vi "UHR-Fleezers Control (fpga, with oscillation) - 10.3.vi"() -> ()   [LabVIEW 2013]
doc: "UHR-Fleezers Instrument Control Code (fpga)"
uses:
  <vilib>/Platform/TimedLoop/XDataNode/timing_clust.ctl
  <vilib>/Platform/TimedLoop/XDataNode/nitl_modes.ctl
  <vilib>/Platform/TimedLoop/XDataNode/wakeup.ctl
  <vilib>/rvi/eio/common/nirviEmuTemplateMethod_errors.vi
  <vilib>/rvi/Emulation/niFpgaSctlEmulationGetInTimedLoop.vi
  <vilib>/rvi/Emulation/niFpgaEmulationReportErrorSimple.vi
  <vilib>/rvi/Emulation/niFpgaGetClockAttributes.vi
  <vilib>/rvi/Emulation/niFpgaCriticalErrorInLSC.vi
  <vilib>/rvi/Emulation/niFpgaProcessEmulError.vi
  <vilib>/rvi/interface/RandomDataEmulation/nirviRandomDataFPGAFIFO.vi
  <vilib>/rvi/interface/RandomDataEmulation/niFpgaRandomDataHandleErrors.vi
  <vilib>/rvi/DataTransferAndStorage/Container/Common/niFpgaContainerExecOnDevCompGetState.vi
  <vilib>/rvi/Memory/Memory_Emulation/nirvimemoryFastEmulationFpgaImpl.vi
  <instcachedir>/0/nirvimemoryFastEmulationFpgaImpl_5FBAB50466BC4C939F684F8805638BFC.lvgen/nirvimemoryFastEmulationFpgaImpl_5FBAB50466BC4C939F684F8805638BFC_002.vi
  <vilib>/rvi/DataTransferAndStorage/Container/Common/niFpgaContainerGetUniqueNameForEmu.vi
  <vilib>/rvi/Memory/Memory_Emulation/niFpgaMemoryEmulationCacheClearOnFirstRun.vi
  <vilib>/rvi/Memory/Memory_Emulation/nirvimemoryEmulationManagerCache_MakeExclusive.vi
  <vilib>/rvi/Memory/Memory_Emulation/niFpgaMemoryEmulationValidateCache.vi
  <vilib>/rvi/Memory/Memory_Emulation/nirvimemoryEmulationManagerCache_ReleaseExclusive.vi
  <vilib>/rvi/Memory/Memory_Emulation/nirvimemoryEmulationManagerCache_InsertValue.vi
  <vilib>/Utility/error.llb/Clear Errors.vi
  <vilib>/rvi/Memory/Memory_Emulation/nirvimemoryEmulationManagerCache_SetValue.vi
  <vilib>/rvi/Emulation/niFpgaSctlEmulationResourceMgr.vi
  <vilib>/rvi/Memory/Memory_Emulation/nirvimemoryEmulationManagerCache_GetValue.vi
  <vilib>/Platform/TimedLoop/XDataNode/XDataNode.xnode
  <vilib>/eio/EIOMethodNode/EIOMethodNode.xnode
  <vilib>/eio/EIONode/EIONode.xnode
  <vilib>/rvi/DataTransferAndStorage/Container/XNode/niFpgaContainer.xnode
  <vilib>/rvi/interface/RandomDataEmulation/nirviRandomDataFpgaReadWriteTemplate.vi
  <vilib>/rvi/Memory/Memory_Emulation/niFpgaMemoryEmulationRefIn.vi
  <vilib>/addons/control/pid/fpga.llb/XNode/niFpgaPID.xnode
  <vilib>/Platform/TimedLoop/XDataNode/XDNodeRunTimeDep.lvlib
panel:
  out "Trap Pos FB Int-Norm Signal":fxp<+/-,16,1> format="%.16g"
  out "Trap Pos FB Int Signal":fxp<+/-,24,9> format="%.18g"
  in  "Tab Control":T1(tab)
  in  "AI1 X Scale":u16
  in  "Trap Pos FB Monitor T1 or T2":bool
  in  "Trap Pos FB Negate Action":bool
  in  "Trap Pos. FB SP":fxp<+/-,16,1>
  in  "Trap Pos. FB Reset":bool
  in  "Trap Pos to FIFO":bool
  in  "AI1 Sets to FIFO":T2={"Set 1"=TRUE, "Set 2"=TRUE, "Set 3"=FALSE}
  in  "N of AI1 Int Acq Sets":i16=2 min=1 max=3 step=1
  out "AI Late Counter":u16
  in  "ai count":u32=400
  out "AI late?":bool
  in  "+ phase":bool
  in  "Phase count adjustment":i16
  out "Relative phase":i16
  in  "AI to FIFO":bool
  out "BD1 Frequency Out 1":u64
  out "BD1 Frequency Out 2":u64
  in  "Force feedback":bool
  out "AI1 X Set 1":fxp<+/-,16,1>
  in  "Trap Pos. FB Gains":T3={"proportional gain (Kc)"=0.0, "integral gain (Kc*Ts/Ti)"=10.0, "derivative gain (Kc*Td/Ts)"=0.0} {"proportional gain (Kc)" format="%.11g"; "integral gain (Kc*Ts/Ti)" format="%.11g"; "derivative gain (Kc*Td/Ts)" format="%.11g"}
  in  "Trap Pos. FB Range":T4={"output high"=0.999969482421875, "output low"=-1.0}
  in  "Trap Pos. FB Mult Factor":i64=2
  in  "Trap Pos. FB Offset Factor":i64
  out "AI1 X Set 2":fxp<+/-,16,1>
  out "Trap Pos FB Action":i64
  out "Trap Pos FIFO Timeout":u16
  out "Trap AI FIFO Timeout":u16
  in  "Trap FIFO Set Timeout":i32
  in  "Trap Pos FB Int Count":u16=100
  in  "Tab Control 2":T5(tab)
  in  "Swap F1 and F2":bool
  in  "Freq or Amp switch first":bool=TRUE
  in  "Cont. Scan":bool
  in  "Abort scan":bool
  in  "Cycles per step":u64
  in  "Scan BD":bool
  in  "Number of scans":u16
  in  "Scan steps":u64
  in  "Scan freq.  increment":i64
  out "Scanning":bool
  in  "Start scan":bool
  in  "OSK Bd 1":bool
  in  "Reset Bd 1":bool
  in  "RD":bool
  in  "PMODE":bool
  in  "OSK Bd 2":bool
  in  "Reset Bd 2":bool
  in  "Direct RF Box \nCommunication":bool
  in  "Data BD 2":u8 format="%08b"
  in  "Data BD 1":u8 format="%08b"
  in  "Address":u8 format="%02x"
  in  "Update Data":bool
  in  "FPGA Controls\n RF Box":bool
  in  "Number Interlace Cycles":u8=2 min=1 max=3
  in  "Interlace Off Parameters":u8=1 min=1 max=3
  in  "Interlace ON/OFF":bool
  out "DIO Relative phase":i16
  in  "Phase count adjustment (DIO)":i16
  in  "+ phase (DIO)":bool
  out "DIO Late Counter":u16
  out "DIO Late?":bool
  in  "DIO count 1 (ticks)":u32=400
  in  "DIO count 2 (ticks)":u32=400
  in  "DIO count 3 (ticks)":u32=400
  out "AI2 Y Sum Set 2":i16
  out "AI2 Y Sum Set 1":i16
  in  "FB Gains Set 1":T6={"proportional gain (Kc)"=10, "integral gain (Kc*Ts/Ti)"=5, "derivative gain (Kc*Td/Ts)"=0}
  in  "FB Setpoint Set 1":i16 min=0 step=1
  in  "FB Reset Set 1":bool
  in  "FB On/Off Set 1":bool
  in  "FB Reset Set 2":bool
  in  "FB On/Off Set 2":bool
  in  "FB Setpoint Set 2":i16 min=0 step=1
  in  "FB Gains Set 2":T6={"proportional gain (Kc)"=10, "integral gain (Kc*Ts/Ti)"=5, "derivative gain (Kc*Td/Ts)"=0}
  in  "FB output range 2":cluster{"output high":i16, "output low":i16}={"output high"=3000, "output low"=0}
  in  "FB output range 1":cluster{"output high":i16, "output low":i16}={"output high"=3000, "output low"=0}
  out "Scan I":u64
  in  "Amp switch delay":u16=5
  in  "Freq switch delay":u16
  in  "Osc trap cont.":bool
  in  "Osc traps":bool
  in  "Initiate trap osc":bool
  in  "Trap osc period (pts)":i16
  in  "N trap osc periods":i16
  in  "Trap 1 osc enable":bool
  in  "Trap 2 osc enable":bool
  in  "Ready Write":bool
  in  "Data":i64
  in  "Address 2":u32
  in  "BD 2 Amplitude 1":u16
  in  "BD 1 Amplitude 1":u16
  in  "BD 2 Frequency 1":u64
  in  "BD 1 Frequency 1":u64
  in  "BD 2 Amplitude 2":u16
  in  "BD 1 Amplitude 2":u16
  in  "BD 2 Frequency 2":u64
  in  "BD 1 Frequency 2":u64
  in  "BD 2 Amplitude 3":u16
  in  "BD 1 Amplitude 3":u16
  in  "BD 2 Frequency 3":u64
  in  "BD 1 Frequency 3":u64
  out "Numeric":i32
  out "AO2 2":i16
  out "AO1 2":i16
  in  "1D or 2D Scan?":bool
  in  "Abort scan (MCL)":bool
  in  "MCL Scan Axis":bool
  in  "Cont. Scan (MCL)":bool
  out "Scan I (MCL)":u64
  in  "Number of scans (MCL)":u16
  out "Scanning MCL":bool
  in  "Scan steps (MCL)":u64
  in  "Cycles per step (MCL)":u64
  in  "Scan freq.  increment (MCL)":i16
  in  "Start scan (MCL)":bool
  in  "AO2":i16
  in  "AO1":i16
  out "MCL Late Counter":u16
  out "MCL Late?":bool
  in  "MCL count":u32=800
  out "MCL Relative Phase":i16
  in  "Phase count adjustment (MCL)":i16
  in  "+ phase (MCL)":bool
  in  "APD Gate Operating Mode":u8 max=2 step=1
  in  "Invert APD Gate":bool
  in  "APD Gate OFF Count":u32=100
  in  "APD Gate ON Count":u32=300
  out "APD 1 Gate Late Counter":u16
  out "APD 1 Gate Late?":bool
  out "APD 1 Gate Relative Phase":i16
  in  "Phase count adjustment (APD 1 Gate)":i16
  in  "+ phase (APD 1 Gate)":bool
  out "APD 2 Counts 0":u32
  out "APD 2 Counts 1":u32
  out "APD 1 Counts 0":u32
  out "APD 1 Counts 1":u32
  out "APD1 out state":bool
  in  "APD 2 AO scale factor":i16=1
  in  "APD 1 AO scale factor":i16=1
  in  "APD to FIFO":bool
  in  "APD Acq Rate Count":u32=20000000
  out "APD Acq Late Counter":u16
  out "APD Acq Late?":bool
  out "APD Acq Relative Phase":i16
  in  "Phase Count Adjustment (APD Acq)":i16
  in  "+ phase (APD Acq)":bool
  in  "Phase count adjustment (APD 2 Gate)":i16
  out "APD 2 Gate Late Counter":u16
  out "APD 2 Gate Late?":bool
  out "APD 2 Gate Relative Phase":i16
  in  "+ phase (APD 2 Gate)":bool
  out "APD2 out state":bool
  in  "Green Filter Flipper":bool
  out "Green FB Signals":T7
  in  "Green FB Count":u32=1200
  out "Green Late Counter":u16
  out "Green FB Late?":bool
  out "Green FB Relative Phase":i16
  in  "Phase count adjustment (Green FB)":i16=10
  in  "+ phase (Green FB)":bool
  out "Green FB Sum":i16
  in  "Green int current ON count adj":u32=150
  in  "Current Out":u16=30000
  in  "Green FB On/Off":bool
  in  "Green FB Setpoint":i16=250 min=0 step=1
  in  "Green FB Gains":T6={"proportional gain (Kc)"=10, "integral gain (Kc*Ts/Ti)"=5, "derivative gain (Kc*Td/Ts)"=0}
  in  "Green FB Reset":bool
  in  "Operating Mode 2":u8=2 max=2 step=1
  in  "Invert GI 2":bool
  in  "Green interlace OFF count 2":u32=900
  in  "Green interlace ON count 2":u32=300
  out "GI Late Counter 2":u16
  out "GI Late? 2":bool
  out "GI Relative phase 2":i16
  in  "Phase count adjustment (GI) 2":i16=20
  in  "+ phase (GI) 2":bool
  in  "Green interlace OFF count":u32=100
  out "GI Relative phase":i16
  in  "Phase count adjustment (GI)":i16
  in  "+ phase (GI)":bool
  out "GI Late?":bool
  in  "Green interlace ON count":u32=300
  out "GI Late Counter":u16
  in  "Invert GI":bool
  in  "Operating Mode":u8 max=2 step=1
  in  "Chassis2/Mod4/AO1":u16
  # "Oscillate Traps\n(e.g., for forced calibration)"
  # "Raster Scan AOD"
  # "Only one of these can be on\nat a time:"
  # "1 (X)"
  # "2 (Y)"
  # "IR Intensity Feedback (RF BD 1)"
  # "AO1 (Y)"
  # "2D"
  # "1D"
  # "AO2 (X)"
  # "APD AO for aligning"
  # "Detection Loop"
  # "Green fluorescent laser digital gate interlacing loop"
  # "0 Forced ON\n1 Forced OFF\n2 Interlacing"
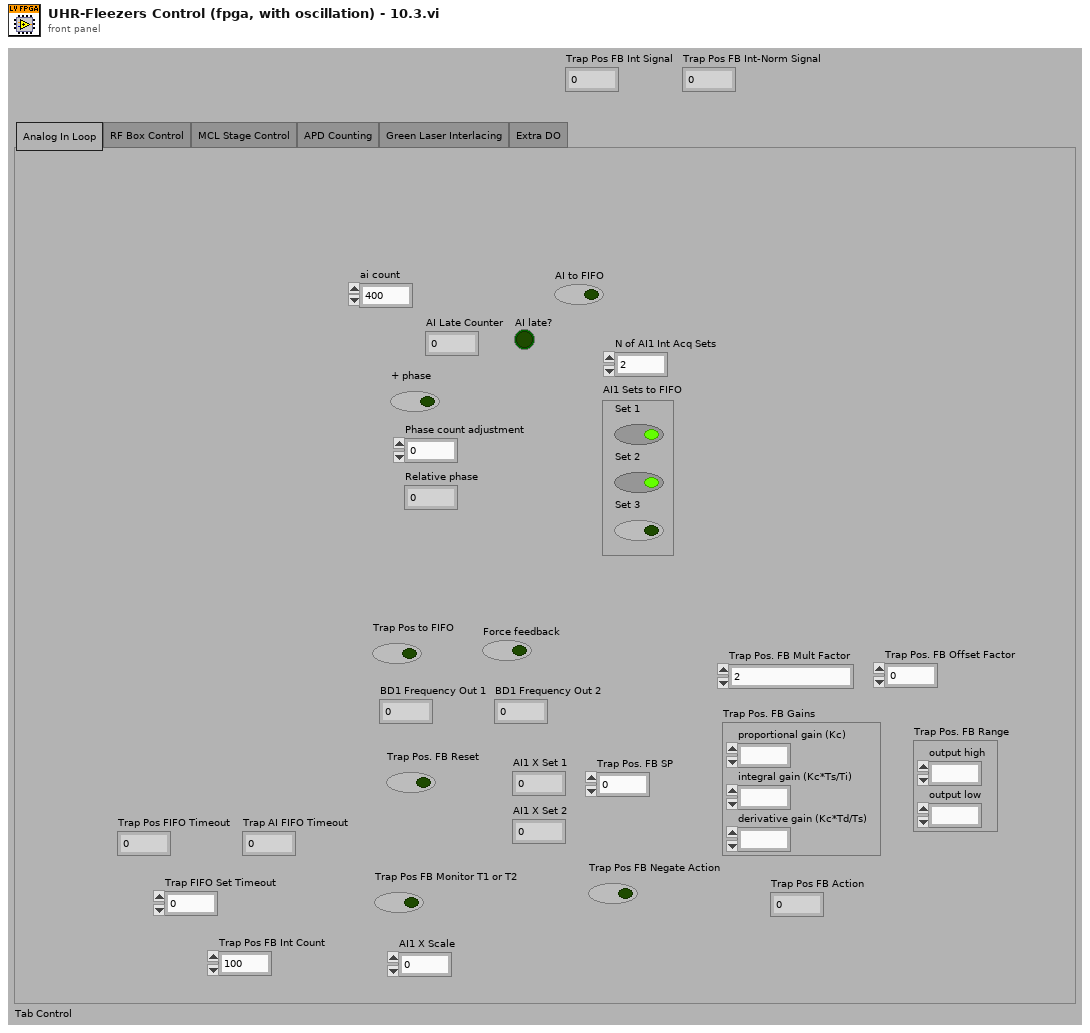
[diagram p1: front panel]
types:
  T1 = enum32{"Analog In Loop", "RF Box Control", "MCL Stage Control", "APD Counting", "Green Laser Interlacing", "Extra DO"}
  T2 = cluster{"Set 1":bool, "Set 2":bool, "Set 3":bool}
  T3 = cluster{"proportional gain (Kc)":fxp<+/-,16,8>, "integral gain (Kc*Ts/Ti)":fxp<+/-,16,8>, "derivative gain (Kc*Td/Ts)":fxp<+/-,16,8>}
  T4 = cluster{"output high":fxp<+/-,16,1>, "output low":fxp<+/-,16,1>}
  T5 = enum32{"Controls", "Interlacing Frequency and Amplitude Values"}
  T6 = cluster{"proportional gain (Kc)":i16, "integral gain (Kc*Ts/Ti)":i16, "derivative gain (Kc*Td/Ts)":i16}
  T7 = cluster{"Green FB Ch 0":i16, "Green FB Ch 1":i16, "Green FB Ch 2":i16}
  T8 = typedef "XDNodeRunTimeDep.lvlib/timing_clust.ctl" = cluster{"Expected End [f-1]":u64, "Actual End [f-1]":u64, "Finished Late? [f-1]":bool, "Expected End [i-1]":u64, "Actual End [i-1]":u64, "Finished Late? [i-1]":bool, "Expected Start [i]":u64, "Actual Start [i]":u64, "Expected Start [f]":u64, "Actual Start [f]":u64, "Source Name":string, "Structure Name":string, "Period":i64, "Deadline":i64, "Offset":i64, "Start":i64, "Priority":i32, "Timeout":i32, "Mode":T9, "Wakeup Reason":T10, "Error":errorcluster, "Source Type":string, "Secondary Source Type":string, "Global End Time":u64, "Global Start Time":u64, "Frame Duration":u64, "Iteration Duration":u64, "Assigned CPU":i32, "I/O Scan Engine Mode":u32}
  T9 = typedef "XDNodeRunTimeDep.lvlib/nitl_modes.ctl" = enum32{"No Change", "Process missed periods, maintain original phase", "Discard missed periods, maintain original phase", "Process missed periods, ignore original phase", "Discard missed periods, ignore original phase"}
  T10 = typedef "XDNodeRunTimeDep.lvlib/wakeup.ctl" = enum32{"Normal", "Aborted", "Asynchronous wakeup", "Timing source error", "Timed loop error", "Timeout"}
  T11 = cluster{"Chassis2/Mod2/AI0":i16, "Chassis2/Mod2/AI1":i16, "Chassis2/Mod2/AI2":i16}
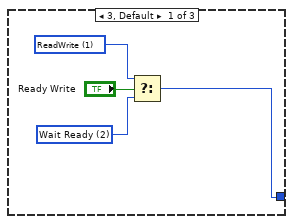
[diagram p2: hidden frame]
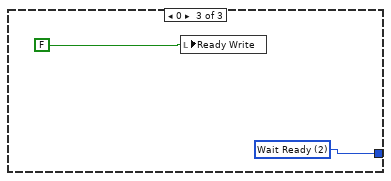
[diagram p3: hidden frame]
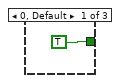
[diagram p4: hidden frame]
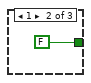
[diagram p5: hidden frame]
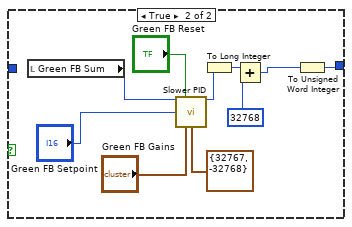
[diagram p6: hidden frame]
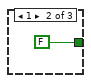
[diagram p7: hidden frame]
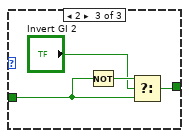
[diagram p8: hidden frame]
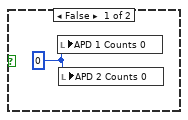
[diagram p9: hidden frame]
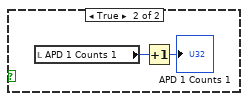
[diagram p11: hidden frame]
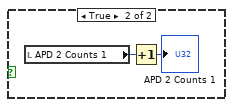
[diagram p12: hidden frame]
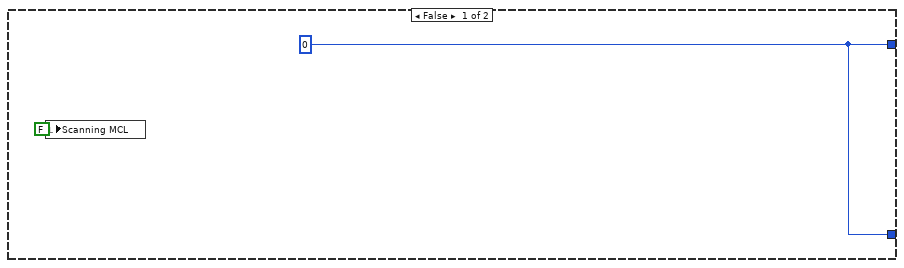
[diagram p13: hidden frame]
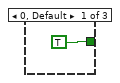
[diagram p14: hidden frame]
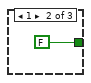
[diagram p15: hidden frame]
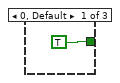
[diagram p16: hidden frame]
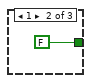
[diagram p17: hidden frame]
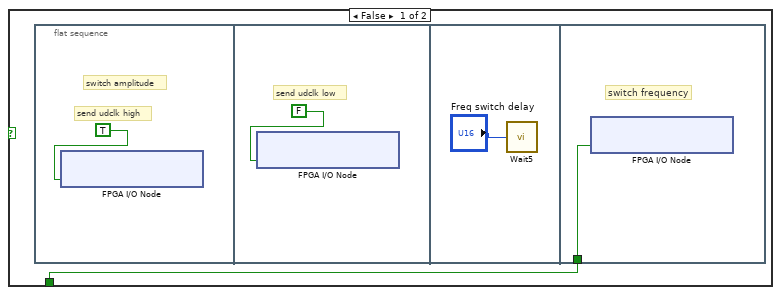
[diagram p20: hidden frame]
diagram:
  w1 = i16 2 items=["UnSet Ready", "ReadWrite", "Wait Ready"]
  w4 = FALSE
  # "timing array current index"
  # "timing array"
  # "timing counter (phase adjusted here)"
  # "late counter"
  n1 = flat-sequence "FPGA initialization to do before running any of the loops" {
    tunnel: [u32 0 ("DIO count 3 (ticks)")] -> w3
    tunnel: [w11] -> _
    frame #0 {
      # "Start up expansion chassis early\nto avoid delays later"
      # "This pin controls udclk on the RF boards.\nWhen initially configuring the boards, this pin needs to be\nconfigured as a high impedance input.  Later it will be switched\nto an output."
      # "Initial setting of DIO data and \naddress to low (before reset).  \nThis needs to happen before the other\ncontrol method loops execute."
      n2 = xnode "FPGA I/O Node"("Connector1/DIO0"=FALSE, "Connector1/DIO1"=FALSE, "Connector1/DIO2"=FALSE, "Connector1/DIO3"=FALSE, "Connector1/DIO4"=FALSE, "Connector1/DIO5"=FALSE, "Connector1/DIO6"=FALSE, "Connector1/DIO7"=FALSE, "Connector1/DIO8"=FALSE, "Connector1/DIO9"=FALSE, "Connector1/DIO10"=FALSE, "Connector1/DIO11"=FALSE, "Connector1/DIO12"=FALSE, "Connector1/DIO13"=FALSE, "Connector1/DIO15"=FALSE, "Connector1/DIO20"=FALSE, "Connector1/DIO21"=FALSE, "Connector1/DIO22"=FALSE, "Connector1/DIO23"=FALSE, "Connector1/DIO24"=FALSE, "Connector1/DIO25"=FALSE, "Connector1/DIO26"=FALSE, "Connector1/DIO27"=FALSE, "Connector1/DIO14"=FALSE) -> ()  [unwired: 24 in, 24 out]
      n3 = xnode "FPGA I/O Method Node"("Enable"=FALSE) -> ()  [unwired: 1 in, 1 out]
      n4 = xnode "FPGA I/O Node"("Chassis2/Mod1/AO0"=u16 0 ("Chassis2/Mod4/AO0")) -> ("Chassis2/Mod2/AI0"=w11:i16)  [unwired: 2 in, 2 out]
    }
  }
  n5 = node-c288() -> (w6:T8)  [unwired: 1 in]
  n6 = timed-loop "RF box board DIO control: control bits" {
    timing: w6 -> [_]
    timing-out: [_] -> w5
    tunnel: [w39] -> _
    tunnel: w3 -> [w39]
    stop <- FALSE stop-if-true
    n7 = xnode "FPGA I/O Node"("Connector1/DIO16"="RD", "Connector1/DIO17"="PMODE", "Connector1/DIO18"="OSK Bd 1", "Connector1/DIO19"="Reset Bd 1", "Connector1/DIO28"="OSK Bd 2", "Connector1/DIO29"="Reset Bd 2") -> ()  [unwired: 6 in, 6 out]
  }
  n8 = local read "AO1"() -> (w8:i16)
  n9 = local read "AO2"() -> (w7:i16)
  n10 = while "APD 1 Counter" {
    tunnel: w3 -> [_]
    stop <- FALSE stop-if-true
    n11 = flat-sequence {
      frame #0 {
        n12 = xnode "FPGA I/O Method Node"("FPGA I/O In"=refnum<k21> "Connector0/DIO0" ("APD 1 DO"), "Timeout"=-1) -> ()  [unwired: 2 out]
      }
      frame #1 {
        n13 = local read "APD1 out state"() -> (w52:bool)
        n14 = case shown="False" w52 {
          frame False {
            n15 = local read "APD 1 Counts 0"() -> (w54:u32)
            n16 = Increment(x=w54) -> (x+1=→"APD 1 Counts 0":u32)
          }
          frame True {
            n17 = local read "APD 1 Counts 1"() -> (w56:u32)
            n18 = Increment(x=w56) -> (x+1=→"APD 1 Counts 1":u32)
          }
        }
      }
    }
  }
  n19 = while "APD 2 Counter" {
    tunnel: w3 -> [_]
    stop <- FALSE stop-if-true
    n20 = flat-sequence {
      frame #0 {
        n21 = xnode "FPGA I/O Method Node"("FPGA I/O In"=refnum<k21> "Connector0/DIO1" ("APD 2 DO"), "Timeout"=-1) -> ()  [unwired: 2 out]
      }
      frame #1 {
        n22 = local read "APD2 out state"() -> (w60:bool)
        n23 = case shown="False" w60 {
          frame False {
            n24 = local read "APD 2 Counts 0"() -> (w62:u32)
            n25 = Increment(x=w62) -> (x+1=→"APD 2 Counts 0":u32)
          }
          frame True {
            n26 = local read "APD 2 Counts 1"() -> (w64:u32)
            n27 = Increment(x=w64) -> (x+1=→"APD 2 Counts 1":u32)
          }
        }
      }
    }
  }
  n28 = while "Control Additional IO (Green laser flip mount)" {
    stop <- FALSE stop-if-true
    n29 = xnode "FPGA I/O Node"("Connector0/DIO3"="Green Filter Flipper", "Chassis2/Mod1/AO1"="Chassis2/Mod4/AO1") -> ()  [unwired: 2 in, 2 out]
    n30 = call "Loop Timer2"("Count(Ticks)"=u32 40000 ("Extra DO Counts")) -> ()  [unwired: 1 out]
  }
  n31 = while "Handshake memory transfer for trap oscillation sin wave data" {
    shift-right: [w70] -> _
    shift-left: w1 -> [w71]
    stop <- FALSE stop-if-true
    # "Write"
    n32 = case shown="1" w71 {
      tunnel: [w74 w79 w80] -> w70
      frame 3, Default {
        w72 = i16 2 items=["UnSet Ready", "ReadWrite", "Wait Ready"]
        w73 = i16 1 items=["UnSet Ready", "ReadWrite", "Wait Ready"]
        n33 = Select(t=w73, s="Ready Write", f=w72) -> (s? t:f=w74:i16)
      }
      frame 1 {
        w79 = i16 0 items=["UnSet Ready", "ReadWrite", "Wait Ready"]
        n34 = xnode ("Memory Write")("Address"="Address 2", "Data"="Data", "Memory In"=refnum<k21> "Trap osc memory") -> ()  [unwired: 1 out]
      }
      frame 0 {
        w80 = i16 2 items=["UnSet Ready", "ReadWrite", "Wait Ready"]
        n35 = local write "Ready Write"(FALSE ("Ready Read")) -> ()
      }
    }
  }
  n36 = while "RF box board direct communication loop" {
    tunnel: w3 -> [_]
    stop <- FALSE stop-if-true
    n37 = case "Whether to use direct communication method (only use one method at a time)" shown="True" "Direct RF Box \nCommunication" {
      frame False {
      }
      frame True {
        n38 = case shown="True" "Update Data" {
          frame False {
          }
          frame True {
            n39 = flat-sequence {
              frame #0 {
                n40 = First Call?() -> (First Call?: T/F=w85:bool)
                n41 = case shown="True" w85 {
                  frame False {
                  }
                  frame True {
                    # "If first time data updated, be sure to set WR high\nbefore setting data and address bits."
                    n42 = flat-sequence {
                      frame #0 {
                        n43 = xnode "FPGA I/O Node"("Connector1/DIO15"=TRUE) -> ()  [unwired: 1 in, 1 out]
                      }
                      frame #1 {
                        n44 = call "Wait"("Count(Ticks)"=u8 40 ("DO Delay 3 (Ticks)")) -> ()  [unwired: 1 out]
                      }
                    }
                  }
                }
              }
              frame #1 {
                n45 = Number To Boolean Array(number="Address") -> (Boolean array=w134:bool[])
                n46 = Number To Boolean Array(number="Data BD 1") -> (Boolean array=w135:bool[])
                n47 = Number To Boolean Array(number="Data BD 2") -> (Boolean array=w104:bool[])
                n48 = Index Array(array=w135, index=7) -> (element=w119:bool)
                n49 = Index Array(array=w135, index=6) -> (element=w118:bool)
                n50 = Index Array(array=w135, index=5) -> (element=w117:bool)
                n51 = Index Array(array=w135, index=4) -> (element=w116:bool)
                n52 = Index Array(array=w135, index=3) -> (element=w115:bool)
                n53 = Index Array(array=w135, index=2) -> (element=w114:bool)
                n54 = Index Array(array=w135, index=1) -> (element=w113:bool)
                n55 = Index Array(array=w135, index=0) -> (element=w112:bool)
                n56 = Index Array(array=w134, index=5) -> (element=w111:bool)
                n57 = Index Array(array=w134, index=4) -> (element=w110:bool)
                n58 = Index Array(array=w134, index=3) -> (element=w109:bool)
                n59 = Index Array(array=w134, index=2) -> (element=w108:bool)
                n60 = Index Array(array=w134, index=1) -> (element=w107:bool)
                n61 = Index Array(array=w134, index=0) -> (element=w106:bool)
                n62 = Index Array(array=w104, index=7) -> (element=w95:bool)
                n63 = Index Array(array=w104, index=6) -> (element=w94:bool)
                n64 = Index Array(array=w104, index=5) -> (element=w93:bool)
                n65 = Index Array(array=w104, index=4) -> (element=w92:bool)
                n66 = Index Array(array=w104, index=3) -> (element=w91:bool)
                n67 = Index Array(array=w104, index=2) -> (element=w90:bool)
                n68 = Index Array(array=w104, index=1) -> (element=w89:bool)
                n69 = Index Array(array=w104, index=0) -> (element=w88:bool)
                n70 = xnode "FPGA I/O Node"("Connector1/DIO0"=w119, "Connector1/DIO1"=w118, "Connector1/DIO2"=w117, "Connector1/DIO3"=w116, "Connector1/DIO4"=w115, "Connector1/DIO5"=w114, "Connector1/DIO6"=w113, "Connector1/DIO7"=w112, "Connector1/DIO8"=w111, "Connector1/DIO9"=w110, "Connector1/DIO10"=w109, "Connector1/DIO11"=w108, "Connector1/DIO12"=w107, "Connector1/DIO13"=w106, "Connector1/DIO20"=w95, "Connector1/DIO21"=w94, "Connector1/DIO22"=w93, "Connector1/DIO23"=w92, "Connector1/DIO24"=w91, "Connector1/DIO25"=w90, "Connector1/DIO26"=w89, "Connector1/DIO27"=w88) -> ()  [unwired: 22 in, 22 out]
              }
              frame #2 {
                # "wait and then apply write signal"
                n71 = call "Wait2"("Count(Ticks)"=u8 40 ("DO Delay 1 (Ticks)")) -> ()  [unwired: 1 out]
              }
              frame #3 {
                # "sending bit low writes data to board buffer"
                n72 = xnode "FPGA I/O Node"("Connector1/DIO15"=FALSE) -> ()  [unwired: 1 in, 1 out]
              }
              frame #4 {
                # "wait then return write signal"
                n73 = call "Wait3"("Count(Ticks)"=u8 40 ("DO Delay 2 (Ticks)")) -> ()  [unwired: 1 out]
              }
              frame #5 {
                # "sending bit high makes ready to\nwrite more data"
                n74 = xnode "FPGA I/O Node"("Connector1/DIO15"=TRUE) -> ()  [unwired: 1 in, 1 out]
              }
            }
          }
        }
      }
    }
  }
  n75 = while "APD 2 Gating" {
    shift-right: [w145] -> _
    shift-left: w3 -> [w150]
    shift-right: [w144] -> _
    shift-left: w4 -> [w142]
    stop <- FALSE stop-if-true
    n76 = flat-sequence {
      tunnel: w150 -> [w153]
      tunnel: [w154] -> w148
      tunnel: [w153] -> w146
      tunnel: [w152] -> w143
      tunnel: w142 -> [w152]
      tunnel: [w157] -> w149
      tunnel: w148 -> [w157]
      tunnel: [w156] -> w147
      tunnel: w146 -> [w156]
      tunnel: w143 -> [w155]
      tunnel: [w175] -> w145
      tunnel: w149 -> [w186]
      tunnel: w147 -> [w184]
      tunnel: [w179] -> w144
      frame #0 {
        n77 = call "Loop Timer8"("Count(Ticks)"=w153) -> ("Tick Count(Ticks)"=w154:u32)
      }
      frame #1 {
        # "(need 4 channels/APD)"
        n78 = xnode "FPGA I/O Node"("Connector1/DIO26"=w155, "Connector1/DIO27"=w155, "Connector1/DIO22"=w155, "Connector1/DIO32"=w155, "Connector1/DIO34"=w155, "Connector1/DIO33"=w155, "Connector1/DIO35"=w155) -> ()  [unwired: 7 in, 7 out]
      }
      frame #2 {
        n79 = local read "APD Gate ON Count"() -> (w168:u32)
        n80 = local read "APD Gate OFF Count"() -> (w167:u32)
        n81 = feedback #1(TRUE) -> (w181:bool)
        n82 = feedback-in #2(w186) -> ()
        n83 = feedback #2(w186) -> (w169:u32)
        n84 = Not(x=w181) -> (.not. x?=w178:bool)
        n85 = feedback-in #1(w178) -> ()
        n86 = Subtract(x=w186, y=w169) -> (x-y=w185:u32)
        n87 = Select(t=w168, s=w178, f=w167) -> (s? t:f=w183:u32)
        n88 = Subtract(x=w185, y=w184) -> (x-y=w160:u32)
        n89 = Subtract(x=w183, y=w160) -> (x-y=w174:u32)
        n90 = Number To Boolean Array(number=w160) -> (Boolean array=w159:bool[])
        n91 = Or Array Elements(Boolean array=w159) -> (logical OR=w158:bool)
        "APD 2 Gate Late?" <- w158
        n92 = Boolean To (0,1)(Boolean="+ phase (APD 2 Gate)") -> (0, 1=w172:i16)
        n93 = Multiply(x=w172, y="Phase count adjustment (APD 2 Gate)") -> (x*y=w170:i16)
        n94 = Boolean To (0,1)(Boolean=w158) -> (0, 1=w165:i16)
        n95 = Add(x=w174, y=w170) -> (x+y=w175:u32)
        n96 = To Unsigned Word Integer(number=w165) -> (unsigned 16bit integer=w162:u16)
        n97 = feedback #3(i16 0) -> (w177:i16)
        n98 = Subtract(x=w177, y=w170) -> (x-y=w176:i16)
        "APD 2 Gate Relative Phase" <- w176
        n99 = feedback-in #3(w176) -> ()
        n100 = feedback #4(u16 0) -> (w163:u16)
        n101 = Add(x=w162, y=w163) -> (x+y=w161:u16)
        "APD 2 Gate Late Counter" <- w161
        n102 = feedback-in #4(w161) -> ()
        n103 = local read "APD Gate Operating Mode"() -> (w166:u8)
        n104 = case shown="2" w166 {
          tunnel: [TRUE FALSE w192] -> w179
          tunnel: w181 -> [_ _ w190]
          frame 0, Default {
          }
          frame 1 {
          }
          frame 2 {
            n105 = local read "Invert APD Gate"() -> (w189:bool)
            n106 = Not(x=w190) -> (.not. x?=w191:bool)
            n107 = Select(t=w191, s=w189, f=w190) -> (s? t:f=w192:bool)
          }
        }
      }
    }
  }
  n108 = while "APD 1 Gating" {
    shift-right: [w196] -> _
    shift-left: w3 -> [w201]
    shift-right: [w195] -> _
    shift-left: w4 -> [w193]
    stop <- FALSE stop-if-true
    n109 = flat-sequence {
      tunnel: w201 -> [w204]
      tunnel: [w205] -> w199
      tunnel: [w204] -> w197
      tunnel: [w203] -> w194
      tunnel: w193 -> [w203]
      tunnel: [w208] -> w200
      tunnel: w199 -> [w208]
      tunnel: [w207] -> w198
      tunnel: w197 -> [w207]
      tunnel: w194 -> [w206]
      tunnel: [w222] -> w196
      tunnel: w200 -> [w237]
      tunnel: w198 -> [w234]
      tunnel: [w226] -> w195
      frame #0 {
        n110 = call "Loop Timer7"("Count(Ticks)"=w204) -> ("Tick Count(Ticks)"=w205:u32)
      }
      frame #1 {
        # "(need 4 channels/APD)"
        n111 = xnode "FPGA I/O Node"("Connector0/DIO8"=w206, "Connector0/DIO9"=w206, "Connector0/DIO10"=w206, "Connector0/DIO11"=w206, "Connector0/DIO4"=w206, "Connector0/DIO5"=w206, "Connector0/DIO6"=w206, "Connector0/DIO7"=w206) -> ()  [unwired: 8 in, 8 out]
      }
      frame #2 {
        n112 = feedback #5(TRUE) -> (w229:bool)
        n113 = feedback-in #6(w237) -> ()
        n114 = feedback #6(w237) -> (w236:u32)
        n115 = Not(x=w229) -> (.not. x?=w225:bool)
        n116 = feedback-in #5(w225) -> ()
        n117 = Subtract(x=w237, y=w236) -> (x-y=w235:u32)
        n118 = Select(t="APD Gate ON Count", s=w225, f="APD Gate OFF Count") -> (s? t:f=w231:u32)
        n119 = Subtract(x=w235, y=w234) -> (x-y=w210:u32)
        n120 = Subtract(x=w231, y=w210) -> (x-y=w221:u32)
        n121 = Number To Boolean Array(number=w210) -> (Boolean array=w211:bool[])
        n122 = Or Array Elements(Boolean array=w211) -> (logical OR=w209:bool)
        "APD 1 Gate Late?" <- w209
        n123 = Boolean To (0,1)(Boolean="+ phase (APD 1 Gate)") -> (0, 1=w219:i16)
        n124 = Boolean To (0,1)(Boolean=w209) -> (0, 1=w216:i16)
        n125 = Multiply(x=w219, y="Phase count adjustment (APD 1 Gate)") -> (x*y=w217:i16)
        n126 = To Unsigned Word Integer(number=w216) -> (unsigned 16bit integer=w213:u16)
        n127 = Add(x=w221, y=w217) -> (x+y=w222:u32)
        n128 = feedback #7(i16 0) -> (w224:i16)
        n129 = Subtract(x=w224, y=w217) -> (x-y=w223:i16)
        "APD 1 Gate Relative Phase" <- w223
        n130 = feedback-in #7(w223) -> ()
        n131 = feedback #8(u16 0) -> (w214:u16)
        n132 = Add(x=w213, y=w214) -> (x+y=w212:u16)
        "APD 1 Gate Late Counter" <- w212
        n133 = feedback-in #8(w212) -> ()
        n134 = case shown="2" "APD Gate Operating Mode" {
          tunnel: [TRUE FALSE w243] -> w226
          tunnel: w229 -> [_ _ w240]
          frame 0, Default {
          }
          frame 1 {
          }
          frame 2 {
            n135 = Not(x=w240) -> (.not. x?=w242:bool)
            n136 = Select(t=w242, s="Invert APD Gate", f=w240) -> (s? t:f=w243:bool)
          }
        }
      }
    }
  }
  n137 = while "DAQ AI set 1" {
    shift-right: [w244] -> _
    shift-left: w3 -> [w249]
    stop <- FALSE stop-if-true
    n138 = flat-sequence {
      tunnel: w249 -> [w259]
      tunnel: [w260] -> w247
      tunnel: [w259] -> w246
      tunnel: [w270] -> w257
      tunnel: [w269] -> w256
      tunnel: [w268] -> w255
      tunnel: [w267] -> w254
      tunnel: [w266] -> w253
      tunnel: [w265] -> w252
      tunnel: [w264] -> w251
      tunnel: [w263] -> w250
      tunnel: [w262] -> w248
      tunnel: w247 -> [w262]
      tunnel: w246 -> [w261]
      tunnel: [w261] -> w245
      tunnel: [w299] -> w244
      tunnel: w257 -> [w327]
      tunnel: w256 -> [w291]
      tunnel: w255 -> [w292]
      tunnel: w254 -> [w326]
      tunnel: w253 -> [w315]
      tunnel: w252 -> [w314]
      tunnel: w251 -> [w313]
      tunnel: w250 -> [w312]
      tunnel: w248 -> [w309]
      tunnel: w245 -> [w306]
      frame #0 {
        n139 = call "Loop Timer3"("Count(Ticks)"=w259) -> ("Tick Count(Ticks)"=w260:u32)
      }
      frame #1 {
        # "detection \nlaser qpd"
        # "sum"
        # "x"
        # "y"
        # "1064 int\nfeedback qpd"
        # "sum"
        # "x"
        # "traps\nqpd"
        # "sum"
        # "y"
        # "x"
        n140 = xnode "FPGA I/O Node"("Connector1/DIO31"=TRUE ("Connector1/DIO33")) -> ("Connector0/AI0"=w270:i16, "Connector0/AI1"=w269:i16, "Connector0/AI2"=w268:i16, "Connector0/AI3"=w267:i16, "Connector0/AI4"=w266:i16, "Connector0/AI5"=w265:i16, "Connector0/AI6"=w264:i16, "Connector0/AI7"=w263:i16)  [unwired: 9 in, 9 out]
      }
      frame #2 {
        w295 = FALSE ("AI to FIFO")
        # "only write specified sets (1 and 2 usually) to FIFO \nif AI to FIFO is true"
        # "Adjust phase after data acquired if button pressed"
        n141 = feedback #9(i16 1) -> (w319:i16)
        n142 = Increment(x=w319) -> (x+1=w325:i16)
        n143 = Scale By Power Of 2(n="AI1 X Scale", x=w291) -> (x*2^n=w289:i16)
        n144 = Greater?(x=w325, y="N of AI1 Int Acq Sets") -> (0:w322:bool)
        n145 = Divide(x=w289, y=w292) -> (x/y=w288:fxp<+/-,16,1>)
        n146 = Select(t=i16 1, s=w322, f=w325) -> (s? t:f=w324:i16)
        n147 = feedback-in #9(w324) -> ()
        n148 = feedback #10(w295) -> (w293:bool)
        n149 = feedback #11(w295) -> (w311:bool)
        n150 = case shown="1, Default" w319 {
          tunnel: w292 -> [w349 w357 _]
          tunnel: "AI1 Sets to FIFO" -> [w353 w361 w367]
          tunnel: [w352 w360 w366] -> w316
          tunnel: ["AI to FIFO" w359 w365] -> w310
          tunnel: w311 -> [_ w359 w365]
          tunnel: ["Trap Pos to FIFO" w358 w364] -> w294
          tunnel: w293 -> [_ w358 w364]
          tunnel: w288 -> [w348 w356 _]
          tunnel: [w347 w354 FALSE] -> w275
          tunnel: [w346 w355 u64 0 ("BD1 Frequency Out 2")] -> w274
          frame 1, Default {
            n151 = Unbundle By Name(w353) -> ("Set 1"=w352:bool)
            n152 = local read "BD1 Frequency Out 1"() -> (w346:u64)
            n153 = Compound Arithmetic op=AND("Trap Pos to FIFO", w352, "AI to FIFO") -> (w347:bool)
            "AI2 Y Sum Set 1" <- w349
            "AI1 X Set 1" <- w348
          }
          frame 2 {
            n154 = Unbundle By Name(w361) -> ("Set 2"=w360:bool)
            n155 = local read "BD1 Frequency Out 2"() -> (w355:u64)
            n156 = Compound Arithmetic op=AND(w358, w360, w359) -> (w354:bool)
            "AI2 Y Sum Set 2" <- w357
            "AI1 X Set 2" <- w356
          }
          frame 3 {
            n157 = Unbundle By Name(w367) -> ("Set 3"=w366:bool)
          }
        }
        n158 = And(x=w316, y=w310) -> (x .and. y?=w318:bool)
        n159 = feedback-in #10(w294) -> ()
        n160 = case shown="True" w318 {
          tunnel: w327 -> [_ w381]
          tunnel: w291 -> [_ w380]
          tunnel: w292 -> [_ w379]
          tunnel: w326 -> [_ w378]
          tunnel: w315 -> [_ w377]
          tunnel: w314 -> [_ w376]
          tunnel: w313 -> [_ w375]
          tunnel: w312 -> [_ w374]
          tunnel: 0 ("DMA buffer timeout") -> [_ w383]
          frame False {
          }
          frame True {
            n161 = Build Array(w381, w380, w379, w378, w377, w376, w375, w374) -> (w382:i16[])
            n162 = for {
              tunnel: w382 -> [w385] mode=indexing
              tunnel: w383 -> [w386]
              tunnel: [w384] -> w372 mode=indexing
              n163 = xnode ("FIFO Write")("Element"=w385, "Timeout"=w386) -> ("Timed Out?"=w384:bool)  [unwired: 1 in, 1 out]
            }
            n164 = Or Array Elements(Boolean array=w372) -> (logical OR=w369:bool)
            n165 = Boolean To (0,1)(Boolean=w369) -> (0, 1=w371:i16)
            n166 = feedback #12(u16 0) -> (w370:u16)
            n167 = Add(x=w371, y=w370) -> (x+y=w368:u16)
            "Trap AI FIFO Timeout" <- w368
            n168 = feedback-in #12(w368) -> ()
          }
        }
        n169 = feedback-in #11(w310) -> ()
        n170 = case shown="True" w275 {
          tunnel: w274 -> [_ w333]
          tunnel: [u8 0 w330] -> w273
          frame False {
          }
          frame True {
            n171 = Split Number(x=w333) -> (hi(x)=w334:u32, lo(x)=w335:u32)
            n172 = Split Number(x=w334) -> (lo(x)=w336:u16)  [unwired: 1 out]
            n173 = Split Number(x=w335) -> (hi(x)=w337:u16, lo(x)=w338:u16)
            n174 = Build Array "BD 1 nu Stack"(w336, w337, w338) -> (w332:u16[])
            n175 = for {
              tunnel: w332 -> [w345] mode=indexing
              shift-right: [w341] -> w330
              shift-left: u8 0 -> [w342]
              n176 = xnode ("FIFO Method Node")("Element"=w345, "Timeout"="Trap FIFO Set Timeout") -> ("Timed Out?"=w344:bool)  [unwired: 1 in, 1 out]
              n177 = Boolean To (0,1)(Boolean=w344) -> (0, 1=w343:i16)
              n178 = To Unsigned Byte Integer(number=w343) -> (unsigned 8bit integer=w340:u8)
              n179 = Add(x=w340, y=w342) -> (x+y=w341:u8)
            }
          }
        }
        n180 = To Unsigned Word Integer(number=w273) -> (unsigned 16bit integer=w272:u16)
        n181 = feedback #13(u16 0) -> (w286:u16)
        n182 = Add(x=w272, y=w286) -> (x+y=w285:u16)
        "Trap Pos FIFO Timeout" <- w285
        n183 = feedback-in #13(w285) -> ()
        n184 = feedback-in #14(w309) -> ()
        n185 = feedback #14(w309) -> (w308:u32)
        n186 = Subtract(x=w309, y=w308) -> (x-y=w307:u32)
        n187 = xnode "I/O Node"("Connector1/DIO31"=FALSE ("Connector1/DIO34")) -> ()  [unwired: 1 in, 1 out]
        n188 = Subtract(x=w307, y=w306) -> (x-y=w277:u32)
        n189 = Boolean To (0,1)(Boolean="+ phase") -> (0, 1=w302:i16)
        n190 = Multiply(x=w302, y="Phase count adjustment") -> (x*y=w296:i16)
        n191 = Subtract(x="ai count", y=w277) -> (x-y=w300:u32)
        n192 = Number To Boolean Array(number=w277) -> (Boolean array=w278:bool[])
        n193 = feedback #15(i16 0) -> (w298:i16)
        n194 = Add(x=w300, y=w296) -> (x+y=w299:u32)
        n195 = Subtract(x=w298, y=w296) -> (x-y=w297:i16)
        "Relative phase" <- w297
        n196 = feedback-in #15(w297) -> ()
        n197 = Or Array Elements(Boolean array=w278) -> (logical OR=w276:bool)
        "AI late?" <- w276
        n198 = Boolean To (0,1)(Boolean=w276) -> (0, 1=w283:i16)
        n199 = To Unsigned Word Integer(number=w283) -> (unsigned 16bit integer=w280:u16)
        n200 = feedback #16(u16 0) -> (w281:u16)
        n201 = Add(x=w280, y=w281) -> (x+y=w279:u16)
        "AI Late Counter" <- w279
        n202 = feedback-in #16(w279) -> ()
      }
    }
  }
  n203 = while "MCL stage control" {
    shift-right: [w402] -> _
    shift-left: w3 -> [w405]
    shift-right: [w395] -> _
    shift-left: w8 -> [w392]
    shift-right: [w394] -> _
    shift-left: w7 -> [w390]
    i -> [w389]
    stop <- FALSE stop-if-true
    n204 = flat-sequence {
      tunnel: w405 -> [w409]
      tunnel: [w410] -> w401
      tunnel: [w409] -> w399
      tunnel: [w408] -> w393
      tunnel: w392 -> [w408]
      tunnel: [w407] -> w391
      tunnel: w390 -> [w407]
      tunnel: w401 -> [w414]
      tunnel: [w414] -> w400
      tunnel: w399 -> [w413]
      tunnel: [w413] -> w398
      tunnel: w393 -> [w412]
      tunnel: w391 -> [w411]
      tunnel: [w412] -> w388
      tunnel: [w411] -> w387
      tunnel: w400 -> [w424]
      tunnel: w398 -> [w423]
      tunnel: [w424] -> w404
      tunnel: [w423] -> w403
      tunnel: [w422] -> w397
      tunnel: [w421] -> w396
      tunnel: w388 -> [w416]
      tunnel: w387 -> [w415]
      tunnel: [w496] -> w402
      tunnel: w404 -> [w503]
      tunnel: w403 -> [w500]
      tunnel: w397 -> [w498]
      tunnel: w396 -> [w497]
      tunnel: [w498] -> w395
      tunnel: [w497] -> w394
      frame #0 {
        n205 = call "Loop Timer5"("Count(Ticks)"=w409) -> ("Tick Count(Ticks)"=w410:u32)
      }
      frame #1 {
        n206 = xnode "FPGA I/O Node"("Connector0/AO1"=w412, "Connector0/AO2"=w411) -> ()  [unwired: 2 in, 2 out]
      }
      frame #2 {
        n207 = local read "Scanning MCL"() -> (w436:bool)
        n208 = Or(x=w436, y="Start scan (MCL)") -> (x .or. y?=w431:bool)
        n209 = Not(x="Abort scan (MCL)") -> (.not. x?=w429:bool)
        n210 = And(x=w429, y=w431) -> (x .and. y?=w428:bool)
        n211 = case "Raster scan" shown="True" w428 {
          tunnel: [w437 w480] -> w433
          tunnel: "Start scan (MCL)" -> [_ w465]
          tunnel: [w437 w441] -> w417
          frame False {
            w437 = i16 0
            n212 = local write "Scanning MCL"(FALSE ("scanning")) -> ()
          }
          frame True {
            w451 = i16 0
            w450 = u64 0
            # "scan incr."
            # "freq. incr. mult."
            # "count steps"
            # "count number of cycles"
            n213 = feedback #17(w450) -> (w477:u64)
            n214 = Select(t=w450, s=w465, f=w477) -> (s? t:f=w479:u64)
            n215 = Increment(x=w479) -> (x+1=w476:u64)
            n216 = Greater?(x="Cycles per step (MCL)", y=w476) -> (0:w460:bool)
            n217 = Select(t=w476, s=w460, f=w450) -> (s? t:f=w475:u64)
            n218 = feedback-in #17(w475) -> ()
            n219 = feedback #18(w450) -> (w474:u64)
            n220 = Select(t=w450, s=w465, f=w474) -> (s? t:f=w469:u64)
            n221 = Increment(x=w469) -> (x+1=w473:u64)
            n222 = Add(x="Scan steps (MCL)", y="Scan steps (MCL)") -> (x+y=w472:u64)
            n223 = Select(t=w469, s=w460, f=w473) -> (s? t:f=w455:u64)
            n224 = Greater?(x=w472, y=w455) -> (0:w454:bool)
            n225 = Select(t=w455, s=w454, f=w450) -> (s? t:f=w470:u64)
            n226 = feedback-in #18(w470) -> ()
            n227 = Equal?(x="Scan steps (MCL)", y=w455) -> (x = y?=w459:bool)
            n228 = Greater?(x="Scan steps (MCL)", y=w469) -> (0:w468:bool)
            n229 = feedback #19(w451) -> (w471:i16)
            n230 = Select(t=w451, s=w465, f=w471) -> (s? t:f=w457:i16)
            n231 = Increment(x=w457) -> (x+1=w467:i16)
            n232 = Decrement(x=w457) -> (x-1=w466:i16)
            n233 = Select(t=w467, s=w468, f=w466) -> (s? t:f=w458:i16)
            n234 = Select(t=w457, s=w459, f=w458) -> (s? t:f=w456:i16)
            n235 = Select(t=w457, s=w460, f=w456) -> (s? t:f=w452:i16)
            n236 = Select(t=w452, s=w454, f=w451) -> (s? t:f=w453:i16)
            n237 = feedback-in #19(w453) -> ()
            n238 = feedback #20(w450) -> (w464:u64)
            n239 = Select(t=w450, s=w465, f=w464) -> (s? t:f=w439:u64)
            n240 = Increment(x=w439) -> (x+1=w461:u64)
            n241 = Select(t=w439, s=w454, f=w461) -> (s? t:f=w440:u64)
            n242 = Greater?(x="Number of scans (MCL)", y=w440) -> (0:w447:bool)
            n243 = Multiply(x="Scan freq.  increment (MCL)", y=w457) -> (x*y=w480:i16)
            n244 = Select(t=TRUE, s="Cont. Scan (MCL)", f=w447) -> (s? t:f=w446:bool)
            "Scanning MCL" <- w446
            n245 = Select(t=w440, s=w446, f=w450) -> (s? t:f=w462:u64)
            n246 = feedback-in #20(w462) -> ()
            n247 = Increment(x=w440) -> (x+1=→"Scan I (MCL)":u64)
            n248 = To Word Integer(number=w439) -> (16bit integer=w442:i16)
            n249 = Multiply(x=w442, y="Scan freq.  increment (MCL)") -> (x*y=w441:i16)
          }
        }
        n250 = Select(t=w417, s="1D or 2D Scan?", f=i16 0) -> (s? t:f=w418:i16)
        n251 = Select(t=w418, s="MCL Scan Axis", f=w433) -> (s? t:f=w432:i16)
        n252 = Select(t=w433, s="MCL Scan Axis", f=w418) -> (s? t:f=w434:i16)
        n253 = Add(x=w432, y="AO2") -> (x+y=w421:i16)
        n254 = Add(x="AO1", y=w434) -> (x+y=w422:i16)
        "AO1 2" <- w416
        "AO2 2" <- w415
      }
      frame #3 {
        n255 = feedback-in #21(w503) -> ()
        n256 = feedback #21(w503) -> (w502:u32)
        n257 = Boolean To (0,1)(Boolean="+ phase (MCL)") -> (0, 1=w494:i16)
        n258 = Subtract(x=w503, y=w502) -> (x-y=w501:u32)
        n259 = Multiply(x=w494, y="Phase count adjustment (MCL)") -> (x*y=w490:i16)
        n260 = Subtract(x=w501, y=w500) -> (x-y=w482:u32)
        n261 = Subtract(x="MCL count", y=w482) -> (x-y=w492:u32)
        n262 = feedback #22(i16 0) -> (w491:i16)
        n263 = Subtract(x=w491, y=w490) -> (x-y=w489:i16)
        "MCL Relative Phase" <- w489
        n264 = feedback-in #22(w489) -> ()
        n265 = Number To Boolean Array(number=w482) -> (Boolean array=w483:bool[])
        n266 = Or Array Elements(Boolean array=w483) -> (logical OR=w481:bool)
        "MCL Late?" <- w481
        n267 = Boolean To (0,1)(Boolean=w481) -> (0, 1=w488:i16)
        n268 = Add(x=w492, y=w490) -> (x+y=w496:u32)
        n269 = To Unsigned Word Integer(number=w488) -> (unsigned 16bit integer=w485:u16)
        n270 = feedback #23(u16 0) -> (w486:u16)
        n271 = Add(x=w485, y=w486) -> (x+y=w484:u16)
        "MCL Late Counter" <- w484
        n272 = feedback-in #23(w484) -> ()
      }
    }
    "Numeric" <- w389
  }
  n273 = while "Control APD data integration - stream to host" {
    shift-right: [w507] -> _
    shift-left: w3 -> [w512]
    stop <- FALSE stop-if-true
    n274 = flat-sequence {
      tunnel: w512 -> [w514]
      tunnel: [w515] -> w510
      tunnel: [w514] -> w508
      tunnel: [w523] -> w511
      tunnel: w510 -> [w523]
      tunnel: [w522] -> w509
      tunnel: w508 -> [w522]
      tunnel: [w521] -> w506
      tunnel: [w520] -> w505
      tunnel: [w557] -> w507
      tunnel: w511 -> [w569]
      tunnel: w509 -> [w566]
      tunnel: w506 -> [w550]
      tunnel: w505 -> [w549]
      frame #0 {
        n275 = call "Loop Timer6"("Count(Ticks)"=w514) -> ("Tick Count(Ticks)"=w515:u32)
      }
      frame #1 {
        n276 = flat-sequence {
          tunnel: [w525] -> w519
          tunnel: w519 -> [w527]
          tunnel: [w529] -> w518
          tunnel: [w528] -> w517
          tunnel: [w527] -> w516
          tunnel: [w535] -> w520
          tunnel: [w536] -> w521
          tunnel: w518 -> [w536]
          tunnel: w517 -> [w535]
          tunnel: w516 -> [w534]
          frame #0 {
            # "use two separate variable so each APD won't\nhave to wait to read"
            n277 = feedback #24(FALSE) -> (w524:bool)
            "APD1 out state" <- w524
            "APD2 out state" <- w524
            n278 = Not(x=w524) -> (.not. x?=w525:bool)
            n279 = feedback-in #24(w525) -> ()
          }
          frame #1 {
            n280 = local read "APD 1 Counts 1"() -> (w533:u32)
            n281 = local read "APD 1 Counts 0"() -> (w532:u32)
            n282 = local read "APD 2 Counts 1"() -> (w531:u32)
            n283 = local read "APD 2 Counts 0"() -> (w530:u32)
            n284 = Select(t=w533, s=w527, f=w532) -> (s? t:f=w529:u32)
            n285 = Select(t=w531, s=w527, f=w530) -> (s? t:f=w528:u32)
          }
          frame #2 {
            n286 = case shown="True" w534 {
              frame False {
                w537 = u32 0 ("APD 1 Counts 0")
                n287 = local write "APD 1 Counts 0"(w537) -> ()
                n288 = local write "APD 2 Counts 0"(w537) -> ()
              }
              frame True {
                w538 = u32 0 ("APD 1 Counts 1")
                n289 = local write "APD 1 Counts 1"(w538) -> ()
                n290 = local write "APD 2 Counts 1"(w538) -> ()
              }
            }
          }
        }
      }
      frame #2 {
        n291 = feedback-in #25(w569) -> ()
        n292 = feedback #25(w569) -> (w568:u32)
        n293 = Subtract(x=w569, y=w568) -> (x-y=w567:u32)
        n294 = Subtract(x=w567, y=w566) -> (x-y=w542:u32)
        n295 = case shown="True" "APD to FIFO" {
          tunnel: w550 -> [_ w572]
          tunnel: w549 -> [_ w570]
          frame False {
          }
          frame True {
            n296 = flat-sequence {
              tunnel: 0 ("Timeout") -> [w574]
              tunnel: w572 -> [w575]
              tunnel: [w574] -> w571
              tunnel: w571 -> [w577]
              tunnel: w570 -> [w576]
              frame #0 {
                n297 = xnode ("FIFO Write")("Element"=w575, "Timeout"=w574) -> ()  [unwired: 1 in, 2 out]
              }
              frame #1 {
                n298 = xnode ("FIFO Write")("Element"=w576, "Timeout"=w577) -> ()  [unwired: 1 in, 2 out]
              }
            }
          }
        }
        n299 = Subtract(x="APD Acq Rate Count", y=w542) -> (x-y=w558:u32)
        n300 = Number To Boolean Array(number=w542) -> (Boolean array=w543:bool[])
        n301 = Or Array Elements(Boolean array=w543) -> (logical OR=w541:bool)
        "APD Acq Late?" <- w541
        n302 = Boolean To (0,1)(Boolean=w541) -> (0, 1=w548:i16)
        n303 = To Unsigned Word Integer(number=w548) -> (unsigned 16bit integer=w545:u16)
        n304 = Boolean To (0,1)(Boolean="+ phase (APD Acq)") -> (0, 1=w554:i16)
        n305 = feedback #26(u16 0) -> (w546:u16)
        n306 = Add(x=w545, y=w546) -> (x+y=w544:u16)
        "APD Acq Late Counter" <- w544
        n307 = feedback-in #26(w544) -> ()
        n308 = Multiply(x=w554, y="Phase Count Adjustment (APD Acq)") -> (x*y=w551:i16)
        n309 = Add(x=w558, y=w551) -> (x+y=w557:u32)
        n310 = feedback #27(i16 0) -> (w556:i16)
        n311 = Subtract(x=w556, y=w551) -> (x-y=w553:i16)
        "APD Acq Relative Phase" <- w553
        n312 = feedback-in #27(w553) -> ()
        n313 = To Word Integer(number=w550) -> (16bit integer=w559:i16)
        n314 = To Word Integer(number=w549) -> (16bit integer=w560:i16)
        n315 = Multiply(x="APD 1 AO scale factor", y=w559) -> (x*y=w540:i16)
        n316 = Multiply(x="APD 2 AO scale factor", y=w560) -> (x*y=w539:i16)
        n317 = xnode "FPGA I/O Node"("Connector0/AO6"=w540, "Connector0/AO7"=w539) -> ()  [unwired: 2 in, 2 out]
      }
    }
  }
  n318 = while "Green fluorescent laser interlacing (DO to IA 532 nm AOM ME amp)." {
    shift-right: [w581] -> _
    shift-left: w3 -> [w586]
    shift-right: [w580] -> _
    shift-left: FALSE -> [w578]
    stop <- FALSE stop-if-true
    n319 = flat-sequence {
      tunnel: w586 -> [w589]
      tunnel: [w590] -> w584
      tunnel: [w589] -> w582
      tunnel: [w588] -> w579
      tunnel: w578 -> [w588]
      tunnel: [w593] -> w585
      tunnel: w584 -> [w593]
      tunnel: [w592] -> w583
      tunnel: w582 -> [w592]
      tunnel: w579 -> [w591]
      tunnel: [w602] -> w581
      tunnel: w585 -> [w622]
      tunnel: w583 -> [w619]
      tunnel: [w611] -> w580
      frame #0 {
        n320 = call "Loop Timer4"("Count(Ticks)"=w589) -> ("Tick Count(Ticks)"=w590:u32)
      }
      frame #1 {
        n321 = xnode "FPGA I/O Node"("Connector1/DIO37"=w591, "Connector1/DIO38"=w591, "Connector1/DIO39"=w591) -> ()  [unwired: 3 in, 3 out]
      }
      frame #2 {
        n322 = feedback-in #28(w622) -> ()
        n323 = feedback #28(w622) -> (w621:u32)
        n324 = Subtract(x=w622, y=w621) -> (x-y=w620:u32)
        n325 = Subtract(x=w620, y=w619) -> (x-y=w595:u32)
        n326 = Number To Boolean Array(number=w595) -> (Boolean array=w596:bool[])
        n327 = Or Array Elements(Boolean array=w596) -> (logical OR=w594:bool)
        "GI Late?" <- w594
        n328 = Boolean To (0,1)(Boolean="+ phase (GI)") -> (0, 1=w607:i16)
        n329 = Multiply(x=w607, y="Phase count adjustment (GI)") -> (x*y=w604:i16)
        n330 = Boolean To (0,1)(Boolean=w594) -> (0, 1=w601:i16)
        n331 = To Unsigned Word Integer(number=w601) -> (unsigned 16bit integer=w598:u16)
        n332 = feedback #29(i16 0) -> (w605:i16)
        n333 = feedback #30(u16 0) -> (w599:u16)
        n334 = Add(x=w598, y=w599) -> (x+y=w597:u16)
        "GI Late Counter" <- w597
        n335 = feedback-in #30(w597) -> ()
        n336 = Subtract(x=w605, y=w604) -> (x-y=w603:i16)
        "GI Relative phase" <- w603
        n337 = feedback-in #29(w603) -> ()
        n338 = feedback #31(TRUE) -> (w614:bool)
        n339 = case shown="2" "Operating Mode" {
          tunnel: [TRUE FALSE w628] -> w611
          tunnel: w614 -> [_ _ w625]
          frame 0, Default {
          }
          frame 1 {
          }
          frame 2 {
            n340 = Not(x=w625) -> (.not. x?=w627:bool)
            n341 = Select(t=w627, s="Invert GI", f=w625) -> (s? t:f=w628:bool)
          }
        }
        n342 = Not(x=w614) -> (.not. x?=w610:bool)
        n343 = Select(t="Green interlace ON count", s=w610, f="Green interlace OFF count") -> (s? t:f=w616:u32)
        n344 = Subtract(x=w616, y=w595) -> (x-y=w608:u32)
        n345 = Add(x=w608, y=w604) -> (x+y=w602:u32)
        n346 = feedback-in #31(w610) -> ()
      }
    }
  }
  n347 = while "Green fluorescent laser interlacing (Current to IA 532 nm AOM ME amp)." {
    shift-right: [w634] -> _
    shift-left: w3 -> [w637]
    shift-right: [w631] -> _
    shift-left: u16 0 -> [w629]
    stop <- FALSE stop-if-true
    n348 = flat-sequence {
      tunnel: w637 -> [w640]
      tunnel: [w641] -> w636
      tunnel: [w640] -> w635
      tunnel: [w639] -> w630
      tunnel: w629 -> [w639]
      tunnel: [w644] -> w633
      tunnel: w636 -> [w644]
      tunnel: [w643] -> w632
      tunnel: w635 -> [w643]
      tunnel: w630 -> [w642]
      tunnel: [w653] -> w634
      tunnel: [w670] -> w631
      tunnel: w633 -> [w683]
      tunnel: w632 -> [w680]
      frame #0 {
        n349 = call "Loop Timer10"("Count(Ticks)"=w640) -> ("Tick Count(Ticks)"=w641:u32)
      }
      frame #1 {
        n350 = xnode "FPGA I/O Node"("Chassis2/Mod1/AO0"=w642) -> ()  [unwired: 1 in, 1 out]
      }
      frame #2 {
        n351 = Subtract(x="Green interlace OFF count 2", y="Green int current ON count adj") -> (x-y=w662:u32)
        n352 = feedback-in #32(w683) -> ()
        n353 = feedback #32(w683) -> (w682:u32)
        n354 = Add(x="Green int current ON count adj", y="Green interlace ON count 2") -> (x+y=w663:u32)
        n355 = Subtract(x=w683, y=w682) -> (x-y=w681:u32)
        n356 = Subtract(x=w681, y=w680) -> (x-y=w646:u32)
        n357 = Number To Boolean Array(number=w646) -> (Boolean array=w647:bool[])
        n358 = Boolean To (0,1)(Boolean="+ phase (GI) 2") -> (0, 1=w659:i16)
        n359 = Or Array Elements(Boolean array=w647) -> (logical OR=w645:bool)
        "GI Late? 2" <- w645
        n360 = Boolean To (0,1)(Boolean=w645) -> (0, 1=w652:i16)
        n361 = Multiply(x=w659, y="Phase count adjustment (GI) 2") -> (x*y=w655:i16)
        n362 = To Unsigned Word Integer(number=w652) -> (unsigned 16bit integer=w648:u16)
        n363 = feedback #33(u16 0) -> (w650:u16)
        n364 = Add(x=w648, y=w650) -> (x+y=w649:u16)
        "GI Late Counter 2" <- w649
        n365 = feedback-in #33(w649) -> ()
        n366 = feedback #34(i16 0) -> (w656:i16)
        n367 = Subtract(x=w656, y=w655) -> (x-y=w654:i16)
        "GI Relative phase 2" <- w654
        n368 = feedback-in #34(w654) -> ()
        n369 = feedback #35(TRUE) -> (w675:bool)
        n370 = case shown="0, Default" "Operating Mode 2" {
          tunnel: [TRUE FALSE w700] -> w664
          tunnel: w675 -> [_ _ w697]
          frame 0, Default {
          }
          frame 1 {
          }
          frame 2 {
            n371 = Not(x=w697) -> (.not. x?=w699:bool)
            n372 = Select(t=w699, s="Invert GI 2", f=w697) -> (s? t:f=w700:bool)
          }
        }
        n373 = And(x=w664, y="Green FB On/Off") -> (x .and. y?=w665:bool)
        n374 = case shown="False" w665 {
          tunnel: "Current Out" -> [w684 _]
          tunnel: [w684 w689] -> w669
          frame False {
          }
          frame True {
            n375 = local read "Green FB Sum"() -> (w685:i16)
            n376 = call "Slower PID.vi"("process variable"=w685, "reset?"="Green FB Reset", "setpoint"="Green FB Setpoint", "PID gains (x 2^8)"="Green FB Gains", "output range"=cluster{"output high":i16, "output low":i16} {"output high"=32767, "output low"=-32768} ("Green FB output range")) -> ("output"=w693:i16)  [unwired: 10 out]
            n377 = To Long Integer(number=w693) -> (32bit integer=w686:i32)
            n378 = Add(x=w686, y=32768) -> (x+y=w688:i32)
            n379 = To Unsigned Word Integer(number=w688) -> (unsigned 16bit integer=w689:u16)
          }
        }
        n380 = Not(x=w675) -> (.not. x?=w672:bool)
        n381 = Select(t=w663, s=w672, f=w662) -> (s? t:f=w677:u32)
        n382 = Subtract(x=w677, y=w646) -> (x-y=w657:u32)
        n383 = Add(x=w657, y=w655) -> (x+y=w653:u32)
        n384 = feedback-in #35(w672) -> ()
        n385 = Boolean To (0,1)(Boolean=w664) -> (0, 1=w671:i16)
        n386 = To Unsigned Word Integer(number=w671) -> (unsigned 16bit integer=w668:u16)
        n387 = Multiply(x=w668, y=w669) -> (x*y=w670:u16)
      }
    }
  }
  n388 = while "Green excitation laser feedback measurement" {
    shift-right: [w701] -> _
    shift-left: w3 -> [w706]
    stop <- FALSE stop-if-true
    n389 = flat-sequence {
      tunnel: w706 -> [w708]
      tunnel: [w709] -> w704
      tunnel: [w708] -> w702
      tunnel: [w716] -> w705
      tunnel: w704 -> [w716]
      tunnel: [w715] -> w703
      tunnel: w702 -> [w715]
      tunnel: [w728] -> w701
      tunnel: w705 -> [w739]
      tunnel: w703 -> [w736]
      frame #0 {
        n390 = call "Loop Timer9"("Count(Ticks)"=w708) -> ("Tick Count(Ticks)"=w709:u32)
      }
      frame #1 {
        n391 = xnode "FPGA I/O Node"("Connector1/DIO35"=TRUE) -> ("Chassis2/Mod2/AI0"=w714:i16, "Chassis2/Mod2/AI1"=w713:i16, "Chassis2/Mod2/AI2"=w710:i16)  [unwired: 4 in, 4 out]
        "Green FB Sum" <- w710
        n392 = Bundle("Chassis2/Mod2/AI0"=w714, "Chassis2/Mod2/AI1"=w713, "Chassis2/Mod2/AI2"=w710) -> (→"Green FB Signals":T11)  [unwired: 1 out]
      }
      frame #2 {
        n393 = feedback-in #36(w739) -> ()
        n394 = feedback #36(w739) -> (w738:u32)
        n395 = Subtract(x=w739, y=w738) -> (x-y=w737:u32)
        n396 = xnode "FPGA I/O Node"("Connector1/DIO35"=FALSE) -> ()  [unwired: 1 in, 1 out]
        n397 = Subtract(x=w737, y=w736) -> (x-y=w718:u32)
        n398 = Subtract(x="Green FB Count", y=w718) -> (x-y=w732:u32)
        n399 = Number To Boolean Array(number=w718) -> (Boolean array=w719:bool[])
        n400 = Or Array Elements(Boolean array=w719) -> (logical OR=w717:bool)
        "Green FB Late?" <- w717
        n401 = Boolean To (0,1)(Boolean="+ phase (Green FB)") -> (0, 1=w730:i16)
        n402 = Boolean To (0,1)(Boolean=w717) -> (0, 1=w724:i16)
        n403 = Multiply(x=w730, y="Phase count adjustment (Green FB)") -> (x*y=w725:i16)
        n404 = Add(x=w732, y=w725) -> (x+y=w728:u32)
        n405 = To Unsigned Word Integer(number=w724) -> (unsigned 16bit integer=w721:u16)
        n406 = feedback #37(i16 0) -> (w727:i16)
        n407 = Subtract(x=w727, y=w725) -> (x-y=w726:i16)
        "Green FB Relative Phase" <- w726
        n408 = feedback-in #37(w726) -> ()
        n409 = feedback #38(u16 0) -> (w722:u16)
        n410 = Add(x=w721, y=w722) -> (x+y=w720:u16)
        "Green Late Counter" <- w720
        n411 = feedback-in #38(w720) -> ()
      }
    }
  }
  n412 = node-c288(w5) -> ()
  n413 = while "RF box board DIO control: parallel communication" {
    shift-right: [w746] -> _
    shift-left: w3 -> [w745]
    shift-right: [w744] -> _
    shift-left: FALSE ("Swap F1 and F2") -> [w743]
    stop <- FALSE stop-if-true
    n414 = flat-sequence {
      tunnel: w743 -> [w750]
      tunnel: w745 -> [w748]
      tunnel: [w750] -> w742
      tunnel: [w749] -> w741
      tunnel: [w748] -> w740
      tunnel: [w756] -> w746
      tunnel: [w755] -> w744
      tunnel: w742 -> [w754]
      tunnel: w741 -> [w752]
      tunnel: w740 -> [w751]
      frame #0 {
        n415 = call "Loop Timer"("Count(Ticks)"=w748) -> ("Tick Count(Ticks)"=w749:u32)
      }
      frame #1 {
        n416 = flat-sequence {
          tunnel: ["FPGA Controls\n RF Box"] -> w753
          tunnel: w754 -> [w757]
          tunnel: [w801] -> w756
          tunnel: [w814] -> w755
          tunnel: w753 -> [w813]
          tunnel: w752 -> [w807]
          tunnel: w751 -> [w804]
          frame #0 {
            n417 = case shown="True" "FPGA Controls\n RF Box" {
              tunnel: w757 -> [_ w759]
              frame False {
              }
              frame True {
                n418 = flat-sequence {
                  tunnel: w759 -> [w765]
                  frame #0 {
                    n419 = First Call?() -> (First Call?: T/F=w760:bool)
                    n420 = case shown="True" w760 {
                      frame False {
                      }
                      frame True {
                        # "If first time data updated, be sure to set WR high and UDCLK low\nbefore setting data and address bits."
                        n421 = xnode "FPGA I/O Method Node"("Enable"=TRUE) -> ("FPGA I/O Out"=w762:refnum<k21>)  [unwired: 1 in]
                        n422 = xnode "FPGA I/O Node"("Connector1/DIO15"=TRUE) -> ()  [unwired: 1 in, 1 out]
                        n423 = xnode "FPGA I/O Node"("I/O Item"=FALSE ("Connector1/DIO30"), "FPGA I/O In"=w762) -> ()  [unwired: 1 out]
                      }
                    }
                  }
                  frame #1 {
                    n424 = case shown="True" "Freq or Amp switch first" {
                      tunnel: w765 -> [w767 w772]
                      frame False {
                        n425 = flat-sequence {
                          tunnel: w767 -> [w771]
                          frame #0 {
                            # "switch amplitude"
                            # "send udclk high"
                            n426 = xnode "FPGA I/O Node"("Connector1/DIO30"=TRUE ("Connector1/DIO15")) -> ()  [unwired: 1 in, 1 out]
                          }
                          frame #1 {
                            # "send udclk low"
                            n427 = xnode "FPGA I/O Node"("Connector1/DIO30"=FALSE ("Connector1/DIO15")) -> ()  [unwired: 1 in, 1 out]
                          }
                          frame #2 {
                            n428 = call "Wait5"("Count(Ticks)"="Freq switch delay") -> ()  [unwired: 1 out]
                          }
                          frame #3 {
                            # "switch frequency"
                            n429 = xnode "FPGA I/O Node"("Connector1/DIO36"=w771) -> ()  [unwired: 1 in, 1 out]
                          }
                        }
                      }
                      frame True {
                        n430 = flat-sequence {
                          tunnel: w772 -> [w773]
                          frame #0 {
                            # "switch frequency"
                            n431 = xnode "FPGA I/O Node"("Connector1/DIO36"=w773) -> ()  [unwired: 1 in, 1 out]
                          }
                          frame #1 {
                            n432 = call "Wait4"("Count(Ticks)"="Amp switch delay") -> ()  [unwired: 1 out]
                          }
                          frame #2 {
                            # "switch amplitude"
                            # "send udclk high"
                            n433 = xnode "FPGA I/O Node"("Connector1/DIO30"=TRUE ("Connector1/DIO15")) -> ()  [unwired: 1 in, 1 out]
                          }
                          frame #3 {
                            # "send udclk low"
                            n434 = xnode "FPGA I/O Node"("Connector1/DIO30"=FALSE ("Connector1/DIO15")) -> ()  [unwired: 1 in, 1 out]
                          }
                        }
                      }
                    }
                  }
                }
              }
            }
          }
          frame #1 {
            # "This is the prior cycle's on time"
            # "increment timing\nindex, reset to 0 if \nend of matrix"
            # "Reset to begginning (1) when number of cycles reached."
            # "timing index"
            # "build byte stacks for writing data\n(must correspond to addresses array constant)"
            # "Timing housekeeping"
            # "Adjust phase if late\n(maintains constant phase relationship between cycles)"
            n435 = feedback #39(u8 0 ("t")) -> (w810:u8)
            n436 = Increment(x=w810) -> (x+1=w853:u8)
            n437 = Increment(x="Number Interlace Cycles") -> (x+1=w848:u8)
            n438 = Equal?(x=w853, y=w848) -> (x = y?=w855:bool)
            n439 = Select(t=u8 1, s=w855, f=w853) -> (s? t:f=w809:u8)
            n440 = feedback-in #39(w809) -> ()
            n441 = Increment(x=w809) -> (x+1=w850:u8)
            n442 = Equal?(x=w850, y=w848) -> (x = y?=w851:bool)
            n443 = Select(t=u8 1, s=w851, f=w850) -> (s? t:f=w847:u8)
            n444 = Select(t=w847, s="Interlace ON/OFF", f="Interlace Off Parameters") -> (s? t:f=w780:u8)
            n445 = feedback-in #40(w807) -> ()
            n446 = feedback #40(w807) -> (w806:u32)
            n447 = Select(t=w809, s="Interlace ON/OFF", f="Interlace Off Parameters") -> (s? t:f=w846:u8)
            n448 = Subtract(x=w807, y=w806) -> (x-y=w805:u32)
            n449 = Subtract "The error"(x=w805, y=w804) -> (x-y=w782:u32)
            n450 = case shown="1, Default" w846 {
              tunnel: ["DIO count 1 (ticks)" "DIO count 2 (ticks)" "DIO count 3 (ticks)"] -> w803
              frame 1, Default {
              }
              frame 2 {
              }
              frame 3 {
              }
            }
            n451 = Number To Boolean Array(number=w782) -> (Boolean array=w783:bool[])
            n452 = Or Array Elements(Boolean array=w783) -> (logical OR=w781:bool)
            "DIO Late?" <- w781
            n453 = Boolean To (0,1)(Boolean=w781) -> (0, 1=w788:i16)
            n454 = To Unsigned Word Integer(number=w788) -> (unsigned 16bit integer=w785:u16)
            n455 = feedback #41(u16 0) -> (w786:u16)
            n456 = Add(x=w785, y=w786) -> (x+y=w784:u16)
            "DIO Late Counter" <- w784
            n457 = feedback-in #41(w784) -> ()
            n458 = Subtract(x=w803, y=w782) -> (x-y=w802:u32)
            n459 = case shown="1, Default" w780 {
              tunnel: [w913 w916] -> w814
              tunnel: [u8 10 u8 4] -> w817
              tunnel: "Swap F1 and F2" -> [w914 w916]
              frame 2 {
                # "F2"
                n460 = Not(x=w914) -> (.not. x?=w913:bool)
              }
              frame 1, Default {
                # "low chooses F1"
                # "F1"
              }
            }
            n461 = feedback #42(i64 0 ("y")) -> (w778:i64)
            n462 = case "Synchronize trap oscillations - always begin/end with trap 1" shown="1, Default" w780 {
              tunnel: [w856 w857 w858] -> w777
              tunnel: w778 -> [w856 w857 _]
              frame 2 {
              }
              frame 3 {
              }
              frame 1, Default {
                n463 = Or(x="Osc traps", y="Initiate trap osc") -> (x .or. y?=w860:bool)
                n464 = case "Trap sine oscillation (or whatever pattern is stored in memory)" shown="True" w860 {
                  tunnel: [i64 0 ("y") w864] -> w858
                  tunnel: "Initiate trap osc" -> [_ w867]
                  frame False {
                  }
                  frame True {
                    w871 = u16 0
                    w869 = -1
                    n465 = local write "Initiate trap osc"(FALSE ("Initiate trap osc")) -> ()
                    n466 = feedback #43(w871) -> (w873:u16)
                    n467 = Select(t=w871, s=w867, f=w873) -> (s? t:f=w872:u16)
                    n468 = Greater Or Equal?(x=w872, y="Trap osc period (pts)") -> (x >= y?=w878:bool)
                    n469 = Or(x=w867, y=w878) -> (x .or. y?=w879:bool)
                    n470 = Select(t=u16 0, s=w879, f=w872) -> (s? t:f=w863:u16)
                    n471 = feedback #44(w869) -> (w870:i32)
                    n472 = Select(t=w869, s=w867, f=w870) -> (s? t:f=w868:i32)
                    n473 = Increment(x=w868) -> (x+1=w875:i32)
                    n474 = Equal?(x=w863, y=u16 0) -> (x = y?=w876:bool)
                    n475 = Increment(x=w863) -> (x+1=w883:u16)
                    n476 = feedback-in #43(w883) -> ()
                    n477 = Select(t=w875, s=w876, f=w868) -> (s? t:f=w874:i32)
                    n478 = feedback-in #44(w874) -> ()
                    n479 = case shown="False" "Osc trap cont." {
                      tunnel: w874 -> [w887 _]
                      frame False {
                        n480 = Greater Or Equal?(x=w887, y="N trap osc periods") -> (x >= y?=w885:bool)
                        n481 = Not(x=w885) -> (.not. x?=w884:bool)
                        n482 = local write "Osc traps"(w884) -> ()
                      }
                      frame True {
                      }
                    }
                    n483 = xnode "Memory Read"("Address"=w863, "Memory In"=refnum<k21> "Trap osc memory") -> ("Data"=w864:i64)  [unwired: 1 out]
                  }
                }
              }
            }
            n484 = case shown="1, Default" w780 {
              tunnel: [w940 w1068 "BD 1 Frequency 3"] -> w843
              tunnel: [w939 "BD 2 Frequency 2" "BD 2 Frequency 3"] -> w832
              tunnel: ["BD 2 Amplitude 1" "BD 2 Amplitude 2" "BD 2 Amplitude 3"] -> w789
              tunnel: [w928 w1070 "BD 1 Amplitude 3"] -> w792
              tunnel: w777 -> [w922 w1064 _]
              frame 1, Default {
                w935 = u64 0 ("f")
                # "Trap 1"
                n485 = local read "Scanning"() -> (w941:bool)
                n486 = case "For position feedback" shown="True" "Force feedback" {
                  tunnel: [i64 0 w959] -> w925
                  frame False {
                  }
                  frame True {
                    w950 = fxp<+/-,24,9> 0.0 ("AI1 X Set 2")
                    w962 = u16 0
                    n487 = local read "AI1 X Set 2"() -> (w956:fxp<+/-,16,1>)
                    n488 = local read "AI1 X Set 1"() -> (w955:fxp<+/-,16,1>)
                    n489 = feedback #45(w962) -> (w963:u16)
                    n490 = Increment(x=w963) -> (x+1=w961:u16)
                    n491 = Select(t=w955, s="Trap Pos FB Monitor T1 or T2", f=w956) -> (s? t:f=w952:fxp<+/-,16,1>)
                    n492 = Greater Or Equal?(x=w961, y="Trap Pos FB Int Count") -> (x >= y?=w953:bool)
                    n493 = Select(t=w962, s=w953, f=w961) -> (s? t:f=w960:u16)
                    n494 = feedback-in #45(w960) -> ()
                    n495 = feedback #46(w950) -> (w951:fxp<+/-,24,9>)
                    n496 = Add(x=w952, y=w951) -> (x+y=w947:fxp<+/-,24,9>)
                    n497 = Select(t=w950, s=w953, f=w947) -> (s? t:f=w949:fxp<+/-,24,9>)
                    n498 = feedback-in #46(w949) -> ()
                    n499 = feedback #47(i64 0) -> (w958:i64)
                    n500 = case shown="True" w953 {
                      tunnel: [w964 w978] -> w959
                      tunnel: w958 -> [w964 _]
                      tunnel: "Trap Pos FB Int Count" -> [_ w966]
                      tunnel: w947 -> [_ w967]
                      frame False {
                      }
                      frame True {
                        n501 = Divide(x=w967, y=w966) -> (x/y=w965:fxp<+/-,16,1>)
                        "Trap Pos FB Int-Norm Signal" <- w965
                        n502 = xnode ("PID")("process variable"=w965, "reset?"="Trap Pos. FB Reset", "setpoint"="Trap Pos. FB SP", "PID gains"="Trap Pos. FB Gains", "output range"="Trap Pos. FB Range") -> ("output"=w976:fxp<+/-,16,1>)
                        n503 = Negate(x=w976) -> (-x=w975:fxp<+/-,17,2>)
                        n504 = Select(t=w975, s="Trap Pos FB Negate Action", f=w976) -> (s? t:f=w972:fxp<+/-,17,2>)
                        n505 = Scale By Power Of 2(n=u32 15, x=u32 1) -> (x*2^n=w969:u32)
                        n506 = Multiply(x=w972, y=w969) -> (x*y=w968:fxp<+/-,17,17>)
                        n507 = To Quad Integer(1:w968) -> (0:w981:i64)
                        "Trap Pos FB Action" <- w981
                        n508 = Multiply(x=w981, y="Trap Pos. FB Mult Factor") -> (x*y=w979:i64)
                        n509 = Add(x=w979, y="Trap Pos. FB Offset Factor") -> (x+y=w978:i64)
                        "Trap Pos FB Int Signal" <- w967
                      }
                    }
                    n510 = feedback-in #47(w959) -> ()
                  }
                }
                n511 = Or(x=w941, y="Start scan") -> (x .or. y?=w933:bool)
                n512 = Not(x="Abort scan") -> (.not. x?=w931:bool)
                n513 = And(x=w931, y=w933) -> (x .and. y?=w930:bool)
                n514 = case "For raster scanning" shown="True" w930 {
                  tunnel: [u64 0 w1053] -> w936
                  tunnel: "Start scan" -> [_ w1038]
                  frame False {
                    n515 = local write "Scanning"(FALSE ("scanning")) -> ()
                  }
                  frame True {
                    w1022 = i64 0
                    w1021 = u64 0
                    # "scan incr."
                    # "freq. incr. mult."
                    # "count steps"
                    # "count number of cycles"
                    n516 = feedback #48(w1021) -> (w1050:u64)
                    n517 = Select(t=w1021, s=w1038, f=w1050) -> (s? t:f=w1052:u64)
                    n518 = Increment(x=w1052) -> (x+1=w1049:u64)
                    n519 = Greater?(x="Cycles per step", y=w1049) -> (0:w1031:bool)
                    n520 = Select(t=w1049, s=w1031, f=w1021) -> (s? t:f=w1048:u64)
                    n521 = feedback-in #48(w1048) -> ()
                    n522 = feedback #49(w1021) -> (w1047:u64)
                    n523 = Select(t=w1021, s=w1038, f=w1047) -> (s? t:f=w1042:u64)
                    n524 = Increment(x=w1042) -> (x+1=w1046:u64)
                    n525 = Add(x="Scan steps", y="Scan steps") -> (x+y=w1045:u64)
                    n526 = Select(t=w1042, s=w1031, f=w1046) -> (s? t:f=w1026:u64)
                    n527 = Greater?(x=w1045, y=w1026) -> (0:w1025:bool)
                    n528 = Select(t=w1026, s=w1025, f=w1021) -> (s? t:f=w1043:u64)
                    n529 = feedback-in #49(w1043) -> ()
                    n530 = Equal?(x="Scan steps", y=w1026) -> (x = y?=w1030:bool)
                    n531 = Greater?(x="Scan steps", y=w1042) -> (0:w1041:bool)
                    n532 = feedback #50(w1022) -> (w1044:i64)
                    n533 = Select(t=w1022, s=w1038, f=w1044) -> (s? t:f=w1028:i64)
                    n534 = Increment(x=w1028) -> (x+1=w1040:i64)
                    n535 = Decrement(x=w1028) -> (x-1=w1039:i64)
                    n536 = Select(t=w1040, s=w1041, f=w1039) -> (s? t:f=w1029:i64)
                    n537 = Select(t=w1028, s=w1030, f=w1029) -> (s? t:f=w1027:i64)
                    n538 = Select(t=w1028, s=w1031, f=w1027) -> (s? t:f=w1023:i64)
                    n539 = Select(t=w1023, s=w1025, f=w1022) -> (s? t:f=w1024:i64)
                    n540 = feedback-in #50(w1024) -> ()
                    n541 = feedback #51(w1021) -> (w1037:u64)
                    n542 = Select(t=w1021, s=w1038, f=w1037) -> (s? t:f=w1033:u64)
                    n543 = Increment(x=w1033) -> (x+1=w1034:u64)
                    n544 = Select(t=w1033, s=w1025, f=w1034) -> (s? t:f=w1032:u64)
                    n545 = Greater?(x="Number of scans", y=w1032) -> (0:w1018:bool)
                    n546 = Multiply(x="Scan freq.  increment", y=w1028) -> (x*y=w1053:i64)
                    n547 = Select(t=TRUE, s="Cont. Scan", f=w1018) -> (s? t:f=w1017:bool)
                    "Scanning" <- w1017
                    n548 = Select(t=w1032, s=w1017, f=w1021) -> (s? t:f=w1035:u64)
                    n549 = feedback-in #51(w1035) -> ()
                    n550 = Increment(x=w1032) -> (x+1=→"Scan I":u64)
                  }
                }
                n551 = case "For intensity feedback" shown="True" "FB On/Off Set 1" {
                  tunnel: "BD 1 Amplitude 1" -> [w1055 _]
                  tunnel: [w1055 w1056] -> w928
                  frame False {
                  }
                  frame True {
                    n552 = local read "AI2 Y Sum Set 1"() -> (w1058:i16)
                    n553 = call "Slower PID.vi"("process variable"=w1058, "reset?"="FB Reset Set 1", "setpoint"="FB Setpoint Set 1", "PID gains (x 2^8)"="FB Gains Set 1", "output range"="FB output range 1") -> ("output"=w1061:i16)  [unwired: 10 out]
                    n554 = To Unsigned Word Integer(number=w1061) -> (unsigned 16bit integer=w1056:u16)
                  }
                }
                n555 = Select(t=w935, s="Scan BD", f=w936) -> (s? t:f=w934:u64)
                n556 = Select(t=w936, s="Scan BD", f=w935) -> (s? t:f=w937:u64)
                n557 = Add(x=w934, y="BD 2 Frequency 1") -> (x+y=w939:u64)
                n558 = Select(t=w922, s="Trap 1 osc enable", f=i64 0) -> (s? t:f=w921:i64)
                n559 = Compound Arithmetic op=ADD(w921, "BD 1 Frequency 1", w925, w937) -> (w940:u64)
                "BD1 Frequency Out 1" <- w940
              }
              frame 2 {
                # "Trap 2"
                n560 = case shown="True" "FB On/Off Set 2" {
                  tunnel: [w1074 w1075] -> w1070
                  tunnel: "BD 1 Amplitude 2" -> [w1074 _]
                  frame False {
                  }
                  frame True {
                    n561 = local read "AI2 Y Sum Set 2"() -> (w1080:i16)
                    n562 = call "Slower PID.vi"("process variable"=w1080, "reset?"="FB Reset Set 2", "setpoint"="FB Setpoint Set 2", "PID gains (x 2^8)"="FB Gains Set 2", "output range"="FB output range 2") -> ("output"=w1077:i16)  [unwired: 10 out]
                    n563 = To Unsigned Word Integer(number=w1077) -> (unsigned 16bit integer=w1075:u16)
                  }
                }
                n564 = Select(t=w1064, s="Trap 2 osc enable", f=i64 0) -> (s? t:f=w1063:i64)
                n565 = Add(x="BD 1 Frequency 2", y=w1063) -> (x+y=w1068:u64)
                "BD1 Frequency Out 2" <- w1068
              }
              frame 3 {
                # "Fluorescence period"
              }
            }
            n566 = Split Number(x=w843) -> (hi(x)=w842:u32, lo(x)=w841:u32)
            n567 = Split Number(x=w832) -> (hi(x)=w837:u32, lo(x)=w836:u32)
            n568 = Split Number(x=w842) -> (lo(x)=w840:u16)  [unwired: 1 out]
            n569 = Split Number(x=w841) -> (hi(x)=w839:u16, lo(x)=w838:u16)
            n570 = Split Number(x=w837) -> (lo(x)=w835:u16)  [unwired: 1 out]
            n571 = Split Number(x=w836) -> (hi(x)=w834:u16, lo(x)=w833:u16)
            n572 = Split Number(x=w792) -> (hi(x)=w794:u8, lo(x)=w793:u8)
            n573 = Split Number(x=w789) -> (hi(x)=w791:u8, lo(x)=w790:u8)
            n574 = Split Number(x=w840) -> (hi(x)=w831:u8, lo(x)=w830:u8)
            n575 = Split Number(x=w839) -> (hi(x)=w829:u8, lo(x)=w828:u8)
            n576 = Split Number(x=w835) -> (hi(x)=w824:u8, lo(x)=w823:u8)
            n577 = Split Number(x=w838) -> (hi(x)=w827:u8, lo(x)=w826:u8)
            n578 = Split Number(x=w834) -> (hi(x)=w822:u8, lo(x)=w821:u8)
            n579 = Split Number(x=w833) -> (hi(x)=w820:u8, lo(x)=w819:u8)
            n580 = Build Array "BD 1 A Stack"(w794, w793) -> (w816:u8[])
            n581 = Build Array "BD 2 A Stack"(w791, w790) -> (w815:u8[])
            n582 = Build Array "BD 1 nu Stack"(w831, w830, w829, w828, w827, w826) -> (w825:u8[])
            n583 = Build Array "BD 2 nu Stack"(w824, w823, w822, w821, w820, w819) -> (w818:u8[])
            n584 = case "If FPGA is controlling (toggling) RF synth" shown="True" w813 {
              tunnel: w825 -> [_ w892]
              tunnel: w818 -> [_ w891]
              tunnel: w817 -> [_ w890]
              tunnel: w816 -> [_ w889]
              tunnel: w815 -> [_ w888]
              frame False {
              }
              frame True {
                # "Write next amp.\n(wait until beginning of next loop iteration to update)"
                n585 = flat-sequence "Update the next F1 and F2 frequency value (the actual frequency won't change until FSK is switched).\nThen load the next amplitude value into buffer, but don't update it until the next cycle." {
                  tunnel: w892 -> [w895]
                  tunnel: w891 -> [w894]
                  tunnel: w890 -> [w893]
                  tunnel: w889 -> [w906]
                  tunnel: w888 -> [w905]
                  frame #0 {
                    n586 = for {
                      tunnel: w895 -> [w901] mode=indexing
                      tunnel: w894 -> [w900] mode=indexing
                      tunnel: w893 -> [w898]
                      i -> [w899]
                      # "Write next freq."
                      n587 = To Unsigned Byte Integer(number=w899) -> (unsigned 8bit integer=w896:u8)
                      n588 = Add(x=w898, y=w896) -> (x+y=w897:u8)
                      n589 = call "write to RF synth bd.vi"("Address Byte"=w897, "BD 2 Byte"=w900, "BD 1 Byte"=w901) -> ()  [unwired: 2 in]
                    }
                  }
                  frame #1 {
                    # "send udclk high"
                    n590 = xnode "FPGA I/O Node"("Connector1/DIO30"=TRUE ("Connector1/DIO15")) -> ()  [unwired: 1 in, 1 out]
                  }
                  frame #2 {
                    n591 = xnode "FPGA I/O Node"("Connector1/DIO30"=FALSE ("Connector1/DIO15")) -> ()  [unwired: 1 in, 1 out]
                  }
                  frame #3 {
                    n592 = for {
                      tunnel: w906 -> [w912] mode=indexing
                      tunnel: w905 -> [w911] mode=indexing
                      tunnel: u8 33 -> [w909]
                      i -> [w910]
                      n593 = To Unsigned Byte Integer(number=w910) -> (unsigned 8bit integer=w907:u8)
                      n594 = Add(x=w909, y=w907) -> (x+y=w908:u8)
                      n595 = call "write to RF synth bd.vi"("Address Byte"=w908, "BD 2 Byte"=w911, "BD 1 Byte"=w912) -> ()  [unwired: 2 in]
                    }
                  }
                }
              }
            }
            n596 = feedback-in #42(w777) -> ()
            n597 = Boolean To (0,1)(Boolean="+ phase (DIO)") -> (0, 1=w799:i16)
            n598 = Multiply(x=w799, y="Phase count adjustment (DIO)") -> (x*y=w795:i16)
            n599 = feedback #52(i16 0) -> (w797:i16)
            n600 = Subtract(x=w797, y=w795) -> (x-y=w796:i16)
            "DIO Relative phase" <- w796
            n601 = feedback-in #52(w796) -> ()
            n602 = Add(x=w802, y=w795) -> (x+y=w801:u32)
          }
        }
      }
    }
  }
